vi "LVIS_Verify.vi"(8 "Error In":errorcluster, 10 "Field Name":string, 11 "Field Value In":string) -> (0 "Error Out":errorcluster, 3 "Field Value Out":string)   [LabVIEW 2015]
doc: "Verifies the field value for a given field name is valid, else throws an error."
uses:
  Globals/LVIS_DcGlobals.vi
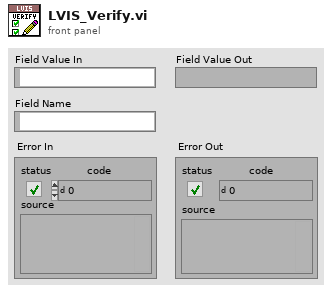
[diagram p1: front panel]
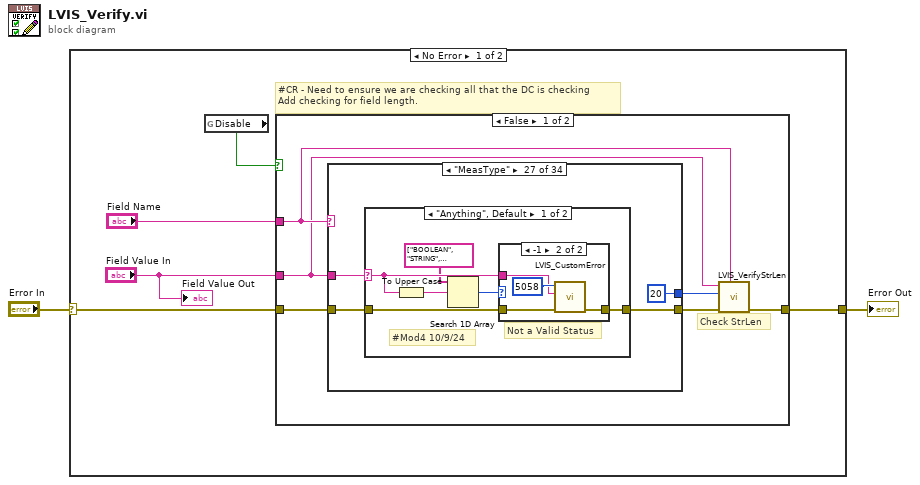
[diagram p0: block diagram]
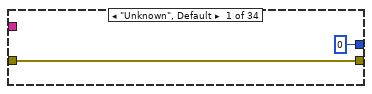
[diagram p2: hidden frame]
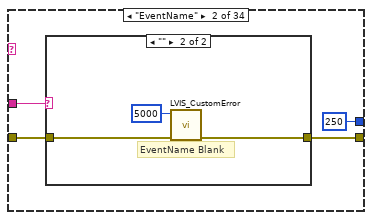
[diagram p3: hidden frame]
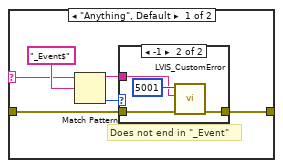
[diagram p4: hidden frame]
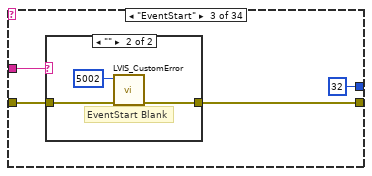
[diagram p6: hidden frame]
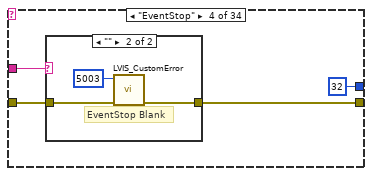
[diagram p8: hidden frame]
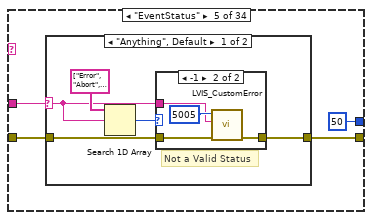
[diagram p10: hidden frame]
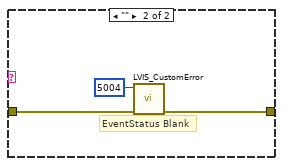
[diagram p12: hidden frame]
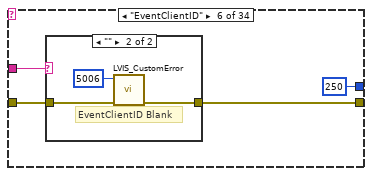
[diagram p13: hidden frame]
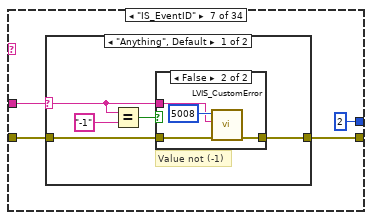
[diagram p15: hidden frame]
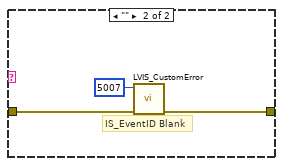
[diagram p17: hidden frame]
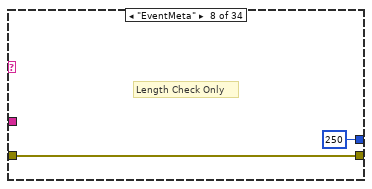
[diagram p18: hidden frame]
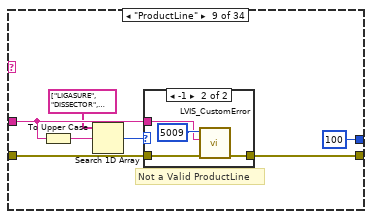
[diagram p19: hidden frame]
diagram:
  n1 = case shown="No Error" "Error In" {
    selector: "Error In" -> [w7 w377]
    tunnel: [w5 w377] -> w1
    frame No Error {
      # "#CR - Need to ensure we are checking all that the DC is checking\nAdd checking for field length."
      n2 = global read "LVIS_DcGlobals.vi" "Disable"() -> (w3:bool)
      n3 = case shown="False" w3 {
        tunnel: w7 -> [w13 w376]
        tunnel: "Field Name" -> [w9 _]
        tunnel: [w11 w376] -> w5
        tunnel: "Field Value In" -> [w8 _]
        frame False {
          # "Check StrLen"
          n4 = case shown="\"MeasType\"" w9 {
            tunnel: w13 -> [w15 w19 w37 w44 w53 w69 w78 w93 w98 w108 w127 w135 w142 w151 w158 w175 w194 w202 w219 w227 w242 w246 w254 w262 w280 w288 w305 w321 w324 w333 w349 w358 w373 w375]
            tunnel: w8 -> [_ w16 w35 w45 w52 w70 w76 _ w97 w109 w125 w133 w143 w150 w159 w174 w193 w201 w217 w225 _ w245 w253 w260 w278 w287 w303 _ w325 w332 w350 w357 _ _]
            tunnel: [w15 w18 w36 w43 w51 w68 w77 w93 w96 w107 w126 w134 w141 w149 w157 w173 w192 w200 w218 w226 w242 w244 w252 w261 w279 w286 w304 w321 w323 w331 w348 w356 w373 w375] -> w12
            tunnel: [0 250 32 32 50 250 2 250 100 50 100 100 50 100 100 250 32 50 250 2 250 250 32 50 250 2 20 75 75 5 75 5 50 250] -> w10
            frame "Unknown", Default {
            }
            frame "EventName" {
              n5 = case shown="\"\"" w16 {
                selector: w16 -> [w21 _]
                tunnel: w19 -> [w24 w33]
                tunnel: [w22 w32] -> w18
                frame "Anything", Default {
                  # "Does not end in \"_Event\""
                  n6 = Match Pattern(string=w21, regular expression="_Event$") -> (before substring=w20:string, offset past match=w23:i32)  [unwired: 1 in, 2 out]
                  n7 = case shown="-1" w23 {
                    tunnel: w24 -> [w26 w30]
                    tunnel: [w26 w28] -> w22
                    tunnel: w20 -> [_ w27]
                    frame 0, Default {
                    }
                    frame -1 {
                      n8 = call "LVIS_CustomError.vi"("error in (no error)"=w30, "Addiitional Info"=w27, "Code"=5001) -> ("error out"=w28:errorcluster)  [unwired: 8 in]
                    }
                  }
                }
                frame "" {
                  # "EventName Blank"
                  n9 = call "LVIS_CustomError.vi"("error in (no error)"=w33, "Code"=5000) -> ("error out"=w32:errorcluster)  [unwired: 9 in]
                }
              }
            }
            frame "EventStart" {
              n10 = case shown="\"\"" w35 {
                tunnel: w37 -> [w38 w41]
                tunnel: [w38 w40] -> w36
                frame "Anything", Default {
                }
                frame "" {
                  # "EventStart Blank"
                  n11 = call "LVIS_CustomError.vi"("error in (no error)"=w41, "Code"=5002) -> ("error out"=w40:errorcluster)  [unwired: 9 in]
                }
              }
            }
            frame "EventStop" {
              n12 = case shown="\"\"" w45 {
                tunnel: w44 -> [w46 w49]
                tunnel: [w46 w48] -> w43
                frame "Anything", Default {
                }
                frame "" {
                  # "EventStop Blank"
                  n13 = call "LVIS_CustomError.vi"("error in (no error)"=w49, "Code"=5003) -> ("error out"=w48:errorcluster)  [unwired: 9 in]
                }
              }
            }
            frame "EventStatus" {
              n14 = case shown="\"Anything\", Default" w52 {
                selector: w52 -> [w54 _]
                tunnel: w53 -> [w58 w66]
                tunnel: [w57 w65] -> w51
                frame "Anything", Default {
                  # "Not a Valid Status"
                  n15 = Search 1D Array(1D array=string[] ["Error", "Abort", "Passed", "Failed", "Logged", "Pending"], element=w54) -> (index of element=w56:i32)  [unwired: 1 in]
                  n16 = case shown="-1" w56 {
                    tunnel: w58 -> [w59 w63]
                    tunnel: [w59 w61] -> w57
                    tunnel: w54 -> [_ w60]
                    frame 0, Default {
                    }
                    frame -1 {
                      n17 = call "LVIS_CustomError.vi"("error in (no error)"=w63, "Addiitional Info"=w60, "Code"=5005) -> ("error out"=w61:errorcluster)  [unwired: 8 in]
                    }
                  }
                }
                frame "" {
                  # "EventStatus Blank"
                  n18 = call "LVIS_CustomError.vi"("error in (no error)"=w66, "Code"=5004) -> ("error out"=w65:errorcluster)  [unwired: 9 in]
                }
              }
            }
            frame "EventClientID" {
              n19 = case shown="\"\"" w70 {
                tunnel: w69 -> [w71 w74]
                tunnel: [w71 w73] -> w68
                frame "Anything", Default {
                }
                frame "" {
                  # "EventClientID Blank"
                  n20 = call "LVIS_CustomError.vi"("error in (no error)"=w74, "Code"=5006) -> ("error out"=w73:errorcluster)  [unwired: 9 in]
                }
              }
            }
            frame "IS_EventID" {
              n21 = case shown="\"Anything\", Default" w76 {
                selector: w76 -> [w79 _]
                tunnel: w78 -> [w83 w91]
                tunnel: [w82 w90] -> w77
                frame "Anything", Default {
                  # "Value not (-1)"
                  n22 = Equal?(x=w79, y="-1") -> (x = y?=w80:bool)
                  n23 = case shown="False" w80 {
                    tunnel: w83 -> [w84 w88]
                    tunnel: [w84 w86] -> w82
                    tunnel: w79 -> [_ w85]
                    frame True {
                    }
                    frame False {
                      n24 = call "LVIS_CustomError.vi"("error in (no error)"=w88, "Addiitional Info"=w85, "Code"=5008) -> ("error out"=w86:errorcluster)  [unwired: 8 in]
                    }
                  }
                }
                frame "" {
                  # "IS_EventID Blank"
                  n25 = call "LVIS_CustomError.vi"("error in (no error)"=w91, "Code"=5007) -> ("error out"=w90:errorcluster)  [unwired: 9 in]
                }
              }
            }
            frame "EventMeta" {
              # "Length Check Only"
            }
            frame "ProductLine" {
              # "Not a Valid ProductLine"
              n26 = To Upper Case(1:w97) -> (0:w99:string)
              n27 = Search 1D Array(1D array=string[] ["LIGASURE", "DISSECTOR", "HARDWARE"], element=w99) -> (index of element=w100:i32)  [unwired: 1 in]
              n28 = case shown="-1" w100 {
                tunnel: w98 -> [w101 w105]
                tunnel: [w101 w103] -> w96
                tunnel: w97 -> [_ w102]
                frame 0, Default {
                }
                frame -1 {
                  n29 = call "LVIS_CustomError.vi"("error in (no error)"=w105, "Addiitional Info"=w102, "Code"=5009) -> ("error out"=w103:errorcluster)  [unwired: 8 in]
                }
              }
            }
            frame "ProcessName" {
              n30 = case shown="\"Anything\", Default" w109 {
                selector: w109 -> [w111 _]
                tunnel: w108 -> [w113 w123]
                tunnel: [w115 w122] -> w107
                frame "Anything", Default {
                  # "Invalid ProcessName"
                  n31 = To Upper Case(1:w111) -> (0:w114:string)
                  n32 = Search 1D Array(1D array=string[] ["MANUFACTURING", "FA_PROCESS", "DEFECT_TRACKING"], element=w114) -> (index of element=w112:i32)  [unwired: 1 in]
                  n33 = case shown="-1" w112 {
                    tunnel: w113 -> [w119 w120]
                    tunnel: [w117 w120] -> w115
                    tunnel: w111 -> [w116 _]
                    frame -1 {
                      n34 = call "LVIS_CustomError.vi"("error in (no error)"=w119, "Addiitional Info"=w116, "Code"=5011) -> ("error out"=w117:errorcluster)  [unwired: 8 in]
                    }
                    frame 0, Default {
                    }
                  }
                }
                frame "" {
                  # "ProcessName Blank"
                  n35 = call "LVIS_CustomError.vi"("error in (no error)"=w123, "Code"=5010) -> ("error out"=w122:errorcluster)  [unwired: 9 in]
                }
              }
            }
            frame "Station" {
              n36 = case shown="\"\"" w125 {
                tunnel: w127 -> [w128 w131]
                tunnel: [w128 w130] -> w126
                frame "Anything", Default {
                }
                frame "" {
                  # "Station Blank"
                  n37 = call "LVIS_CustomError.vi"("error in (no error)"=w131, "Code"=5012) -> ("error out"=w130:errorcluster)  [unwired: 9 in]
                }
              }
            }
            frame "Operator" {
              n38 = case shown="\"\"" w133 {
                tunnel: w135 -> [w136 w139]
                tunnel: [w136 w138] -> w134
                frame "Anything", Default {
                }
                frame "" {
                  # "Operator Blank"
                  n39 = call "LVIS_CustomError.vi"("error in (no error)"=w139, "Code"=5013) -> ("error out"=w138:errorcluster)  [unwired: 9 in]
                }
              }
            }
            frame "SN" {
              n40 = case shown="\"\"" w143 {
                tunnel: w142 -> [w144 w147]
                tunnel: [w144 w146] -> w141
                frame "Anything", Default {
                }
                frame "" {
                  # "SN Blank"
                  n41 = call "LVIS_CustomError.vi"("error in (no error)"=w147, "Code"=5014) -> ("error out"=w146:errorcluster)  [unwired: 9 in]
                }
              }
            }
            frame "Model" {
              n42 = case shown="\"\"" w150 {
                tunnel: w151 -> [w152 w155]
                tunnel: [w152 w154] -> w149
                frame "Anything", Default {
                }
                frame "" {
                  # "Model Blank"
                  n43 = call "LVIS_CustomError.vi"("error in (no error)"=w155, "Code"=5015) -> ("error out"=w154:errorcluster)  [unwired: 9 in]
                }
              }
            }
            frame "Manufacturer" {
              n44 = case shown="\"Anything\", Default" w159 {
                selector: w159 -> [w160 _]
                tunnel: w158 -> [w164 w172]
                tunnel: [w163 w171] -> w157
                frame "Anything", Default {
                  # "Invalid Manufacturer"
                  n45 = Equal?(x="Medtronic" ("y"), y=w160) -> (x = y?=w161:bool)
                  n46 = case shown="False" w161 {
                    tunnel: w164 -> [w165 w169]
                    tunnel: [w165 w167] -> w163
                    tunnel: w160 -> [_ w166]
                    frame True {
                    }
                    frame False {
                      n47 = call "LVIS_CustomError.vi"("error in (no error)"=w169, "Addiitional Info"=w166, "Code"=5017) -> ("error out"=w167:errorcluster)  [unwired: 8 in]
                    }
                  }
                }
                frame "" {
                  # "Manufacturer Blank"
                  n48 = call "LVIS_CustomError.vi"("error in (no error)"=w172, "Code"=5016) -> ("error out"=w171:errorcluster)  [unwired: 9 in]
                }
              }
            }
            frame "TestName" {
              n49 = case shown="\"Anything\", Default" w174 {
                selector: w174 -> [w178 _]
                tunnel: w175 -> [w181 w190]
                tunnel: [w179 w189] -> w173
                frame "Anything", Default {
                  # "Does not end in \"_Tests\""
                  n50 = Match Pattern(string=w178, regular expression="_Tests$") -> (before substring=w177:string, offset past match=w180:i32)  [unwired: 1 in, 2 out]
                  n51 = case shown="-1" w180 {
                    tunnel: w181 -> [w183 w187]
                    tunnel: [w183 w185] -> w179
                    tunnel: w177 -> [_ w184]
                    frame 0, Default {
                    }
                    frame -1 {
                      n52 = call "LVIS_CustomError.vi"("error in (no error)"=w187, "Addiitional Info"=w184, "Code"=5031) -> ("error out"=w185:errorcluster)  [unwired: 8 in]
                    }
                  }
                }
                frame "" {
                  # "TestName Blank"
                  n53 = call "LVIS_CustomError.vi"("error in (no error)"=w190, "Code"=5030) -> ("error out"=w189:errorcluster)  [unwired: 9 in]
                }
              }
            }
            frame "TestDateTime" {
              n54 = case shown="\"\"" w193 {
                tunnel: w194 -> [w195 w198]
                tunnel: [w195 w197] -> w192
                frame "Anything", Default {
                }
                frame "" {
                  # "TestDateTime Blank"
                  n55 = call "LVIS_CustomError.vi"("error in (no error)"=w198, "Code"=5032) -> ("error out"=w197:errorcluster)  [unwired: 9 in]
                }
              }
            }
            frame "TestStatus" {
              n56 = case shown="\"Anything\", Default" w201 {
                selector: w201 -> [w203 _]
                tunnel: w202 -> [w207 w215]
                tunnel: [w206 w214] -> w200
                frame "Anything", Default {
                  # "Not a Valid Status"
                  n57 = Search 1D Array(1D array=string[] ["Error", "Abort", "Passed", "Failed", "Logged", "Pending"], element=w203) -> (index of element=w205:i32)  [unwired: 1 in]
                  n58 = case shown="-1" w205 {
                    tunnel: w207 -> [w208 w212]
                    tunnel: [w208 w210] -> w206
                    tunnel: w203 -> [_ w209]
                    frame 0, Default {
                    }
                    frame -1 {
                      n59 = call "LVIS_CustomError.vi"("error in (no error)"=w212, "Addiitional Info"=w209, "Code"=5034) -> ("error out"=w210:errorcluster)  [unwired: 8 in]
                    }
                  }
                }
                frame "" {
                  # "TestStatus Blank"
                  n60 = call "LVIS_CustomError.vi"("error in (no error)"=w215, "Code"=5033) -> ("error out"=w214:errorcluster)  [unwired: 9 in]
                }
              }
            }
            frame "TestClientID" {
              n61 = case shown="\"\"" w217 {
                tunnel: w219 -> [w220 w223]
                tunnel: [w220 w222] -> w218
                frame "Anything", Default {
                }
                frame "" {
                  # "TestClientID Blank"
                  n62 = call "LVIS_CustomError.vi"("error in (no error)"=w223, "Code"=5035) -> ("error out"=w222:errorcluster)  [unwired: 9 in]
                }
              }
            }
            frame "IS_TestID" {
              n63 = case shown="\"Anything\", Default" w225 {
                selector: w225 -> [w228 _]
                tunnel: w227 -> [w232 w240]
                tunnel: [w231 w239] -> w226
                frame "Anything", Default {
                  # "Value not (-1)"
                  n64 = Equal?(x=w228, y="-1") -> (x = y?=w229:bool)
                  n65 = case shown="False" w229 {
                    tunnel: w232 -> [w233 w237]
                    tunnel: [w233 w235] -> w231
                    tunnel: w228 -> [_ w234]
                    frame True {
                    }
                    frame False {
                      n66 = call "LVIS_CustomError.vi"("error in (no error)"=w237, "Addiitional Info"=w234, "Code"=5037) -> ("error out"=w235:errorcluster)  [unwired: 8 in]
                    }
                  }
                }
                frame "" {
                  # "IS_TestID Blank"
                  n67 = call "LVIS_CustomError.vi"("error in (no error)"=w240, "Code"=5036) -> ("error out"=w239:errorcluster)  [unwired: 9 in]
                }
              }
            }
            frame "TestMeta" {
              # "Length Check Only"
            }
            frame "MeasName" {
              n68 = case shown="\"\"" w245 {
                tunnel: w246 -> [w247 w250]
                tunnel: [w247 w249] -> w244
                frame "Anything", Default {
                }
                frame "" {
                  # "MeasName Blank"
                  n69 = call "LVIS_CustomError.vi"("error in (no error)"=w250, "Code"=5050) -> ("error out"=w249:errorcluster)  [unwired: 9 in]
                }
              }
            }
            frame "MeasDateTime" {
              n70 = case shown="\"\"" w253 {
                tunnel: w254 -> [w255 w258]
                tunnel: [w255 w257] -> w252
                frame "Anything", Default {
                }
                frame "" {
                  # "MeasDateTime Blank"
                  n71 = call "LVIS_CustomError.vi"("error in (no error)"=w258, "Code"=5051) -> ("error out"=w257:errorcluster)  [unwired: 9 in]
                }
              }
            }
            frame "MeasStatus" {
              n72 = case shown="\"Anything\", Default" w260 {
                selector: w260 -> [w265 _]
                tunnel: w262 -> [w268 w276]
                tunnel: [w267 w275] -> w261
                frame "Anything", Default {
                  # "Not a Valid Status"
                  n73 = To Upper Case(1:w265) -> (0:w263:string)
                  n74 = Search 1D Array(1D array=string[] ["ERROR", "ABORT", "PASSED", "FAILED", "LOGGED", "DERIVE"], element=w263) -> (index of element=w266:i32)  [unwired: 1 in]
                  n75 = case shown="-1" w266 {
                    tunnel: w268 -> [w269 w273]
                    tunnel: [w269 w271] -> w267
                    tunnel: w265 -> [_ w270]
                    frame 0, Default {
                    }
                    frame -1 {
                      n76 = call "LVIS_CustomError.vi"("error in (no error)"=w273, "Addiitional Info"=w270, "Code"=5053) -> ("error out"=w271:errorcluster)  [unwired: 8 in]
                    }
                  }
                }
                frame "" {
                  # "MeasStatus Blank"
                  n77 = call "LVIS_CustomError.vi"("error in (no error)"=w276, "Code"=5052) -> ("error out"=w275:errorcluster)  [unwired: 9 in]
                }
              }
            }
            frame "MeasClientID" {
              n78 = case shown="\"\"" w278 {
                tunnel: w280 -> [w281 w284]
                tunnel: [w281 w283] -> w279
                frame "Anything", Default {
                }
                frame "" {
                  # "MeasClientID Blank"
                  n79 = call "LVIS_CustomError.vi"("error in (no error)"=w284, "Code"=5054) -> ("error out"=w283:errorcluster)  [unwired: 9 in]
                }
              }
            }
            frame "IS_MeasID" {
              n80 = case shown="\"Anything\", Default" w287 {
                selector: w287 -> [w289 _]
                tunnel: w288 -> [w293 w301]
                tunnel: [w292 w300] -> w286
                frame "Anything", Default {
                  # "Value not (-1)"
                  n81 = Equal?(x=w289, y="-1") -> (x = y?=w290:bool)
                  n82 = case shown="False" w290 {
                    tunnel: w293 -> [w294 w298]
                    tunnel: [w294 w296] -> w292
                    tunnel: w289 -> [_ w295]
                    frame True {
                    }
                    frame False {
                      n83 = call "LVIS_CustomError.vi"("error in (no error)"=w298, "Addiitional Info"=w295, "Code"=5056) -> ("error out"=w296:errorcluster)  [unwired: 8 in]
                    }
                  }
                }
                frame "" {
                  # "IS_MeasID Blank"
                  n84 = call "LVIS_CustomError.vi"("error in (no error)"=w301, "Code"=5055) -> ("error out"=w300:errorcluster)  [unwired: 9 in]
                }
              }
            }
            frame "MeasType" {
              n85 = case shown="\"Anything\", Default" w303 {
                selector: w303 -> [w308 _]
                tunnel: w305 -> [w311 w319]
                tunnel: [w310 w318] -> w304
                frame "Anything", Default {
                  # "#Mod4 10/9/24"
                  # "Not a Valid Status"
                  n86 = To Upper Case(1:w308) -> (0:w307:string)
                  n87 = Search 1D Array(1D array=string[] ["BOOLEAN", "STRING", "NUMBER", "LOGGED"], element=w307) -> (index of element=w309:i32)  [unwired: 1 in]
                  n88 = case shown="-1" w309 {
                    tunnel: w311 -> [w312 w316]
                    tunnel: [w312 w314] -> w310
                    tunnel: w308 -> [_ w313]
                    frame 0, Default {
                    }
                    frame -1 {
                      n89 = call "LVIS_CustomError.vi"("error in (no error)"=w316, "Addiitional Info"=w313, "Code"=5058) -> ("error out"=w314:errorcluster)  [unwired: 8 in]
                    }
                  }
                }
                frame "" {
                  # "EventType Blank"
                  n90 = call "LVIS_CustomError.vi"("error in (no error)"=w319, "Code"=5057) -> ("error out"=w318:errorcluster)  [unwired: 9 in]
                }
              }
            }
            frame "MeasValue" {
              # "Length Check Only"
            }
            frame "LL" {
              n91 = case shown="\"\"" w325 {
                tunnel: w324 -> [w326 w329]
                tunnel: [w326 w328] -> w323
                frame "Anything", Default {
                }
                frame "" {
                  # "LL Blank"
                  n92 = call "LVIS_CustomError.vi"("error in (no error)"=w329, "Code"=5059) -> ("error out"=w328:errorcluster)  [unwired: 9 in]
                }
              }
            }
            frame "LL Comp" {
              n93 = case shown="\"Anything\", Default" w332 {
                selector: w332 -> [w335 _]
                tunnel: w333 -> [w338 w346]
                tunnel: [w337 w345] -> w331
                frame "Anything", Default {
                  # "Not a Valid Status"
                  n94 = Search 1D Array(1D array=string[] ["GT", "GE", "EQ", "NE"], element=w335) -> (index of element=w336:i32)  [unwired: 1 in]
                  n95 = case shown="-1" w336 {
                    tunnel: w338 -> [w339 w343]
                    tunnel: [w339 w341] -> w337
                    tunnel: w335 -> [_ w340]
                    frame 0, Default {
                    }
                    frame -1 {
                      n96 = call "LVIS_CustomError.vi"("error in (no error)"=w343, "Addiitional Info"=w340, "Code"=5061) -> ("error out"=w341:errorcluster)  [unwired: 8 in]
                    }
                  }
                }
                frame "" {
                  # "LL Comp Blank"
                  n97 = call "LVIS_CustomError.vi"("error in (no error)"=w346, "Code"=5060) -> ("error out"=w345:errorcluster)  [unwired: 9 in]
                }
              }
            }
            frame "HL" {
              n98 = case shown="\"\"" w350 {
                tunnel: w349 -> [w351 w354]
                tunnel: [w351 w353] -> w348
                frame "Anything", Default {
                }
                frame "" {
                  # "HL Blank"
                  n99 = call "LVIS_CustomError.vi"("error in (no error)"=w354, "Code"=5062) -> ("error out"=w353:errorcluster)  [unwired: 9 in]
                }
              }
            }
            frame "HL Comp" {
              n100 = case shown="\"Anything\", Default" w357 {
                selector: w357 -> [w360 _]
                tunnel: w358 -> [w363 w371]
                tunnel: [w362 w370] -> w356
                frame "Anything", Default {
                  # "Not a Valid Status"
                  n101 = Search 1D Array(1D array=string[] ["EQ", "NE", "LE", "LT"], element=w360) -> (index of element=w361:i32)  [unwired: 1 in]
                  n102 = case shown="-1" w361 {
                    tunnel: w363 -> [w364 w368]
                    tunnel: [w364 w366] -> w362
                    tunnel: w360 -> [_ w365]
                    frame 0, Default {
                    }
                    frame -1 {
                      n103 = call "LVIS_CustomError.vi"("error in (no error)"=w368, "Addiitional Info"=w365, "Code"=5064) -> ("error out"=w366:errorcluster)  [unwired: 8 in]
                    }
                  }
                }
                frame "" {
                  # "HL Comp Blank"
                  n104 = call "LVIS_CustomError.vi"("error in (no error)"=w371, "Code"=5063) -> ("error out"=w370:errorcluster)  [unwired: 9 in]
                }
              }
            }
            frame "Units" {
              # "Length check only"
            }
            frame "MeasMeta" {
              # "Length check only"
            }
          }
          n105 = call "LVIS_VerifyStrLen.vi"("Field Name"=w9, "Error In"=w12, "Max StrLen"=w10, "Field Value In"=w8) -> ("Error Out"=w11:errorcluster)  [unwired: 7 in]
        }
        frame True {
          # "The Data Commander has been disabled"
        }
      }
      "Field Value Out" <- "Field Value In"
    }
    frame Error {
    }
  }
  "Error Out" <- w1
